vi "Main Test App.vi"() -> ()   [LabVIEW 2010]
panel:
  out "Limit Test Passed?":bool
  in  "Lower LED Limit (V)":dbl=1.63
  in  "Upper LED Limit (V)":dbl=1.635
  out "LED Test Passed?":bool
  in  "Filter Error Limits (+/- V)":dbl=0.06
  out "Limit Test Results":cluster{dbl[], dbl[]}[](graph)=[{[1000.0, 9166.666666666668, 17333.333333333336, 25500.0, 33666.66666666667, 41833.333333333336, 50000.0], [0.8109999999999999, 0.7375, 0.6639999999999999, 0.5905, 0.5169999999999999, 0.44349999999999995, 0.37]}, {[1000.0, 9166.666666666668, 17333.333333333336, 25500.0, 33666.66666666667, 41833.333333333336, 50000.0], [0.7794851199823166, 0.7105386097097423, 0.600359382509452, 0.5104585406834482, 0.4415120304108739, 0.3921679593334433, 0.3549909194805846]}, {[1000.0, 9166.666666666668, 17333.333333333336, 25500.0, 33666.66666666667, 41833.333333333336, 50000.0], [0.6910000000000001, 0.6174999999999999, 0.544, 0.4705, 0.39699999999999996, 0.32349999999999995, 0.25]}]
  in  "Select XML Config File":u16(ring)=2 items=["PXI Mod Instr Config 081226.xml", "Legacy Instr Config 081226.xml", "Simulated Instruments.xml"]
  out "Actual LED Voltage (V)":dbl
  in  "error in (no error)":errorcluster
  out "error out":errorcluster
  in  "Number of Steps":i32=7
  in  "Start Frequency (>1K Hz)":dbl=1000.0
  in  "Stop Frquency (<50k Hz)":dbl=50000.0
  # "Filter Limit Test Results"
  # "Filter Limit Test Parameters"
  # "LED Test Parameters"
  # "LED Test Results"
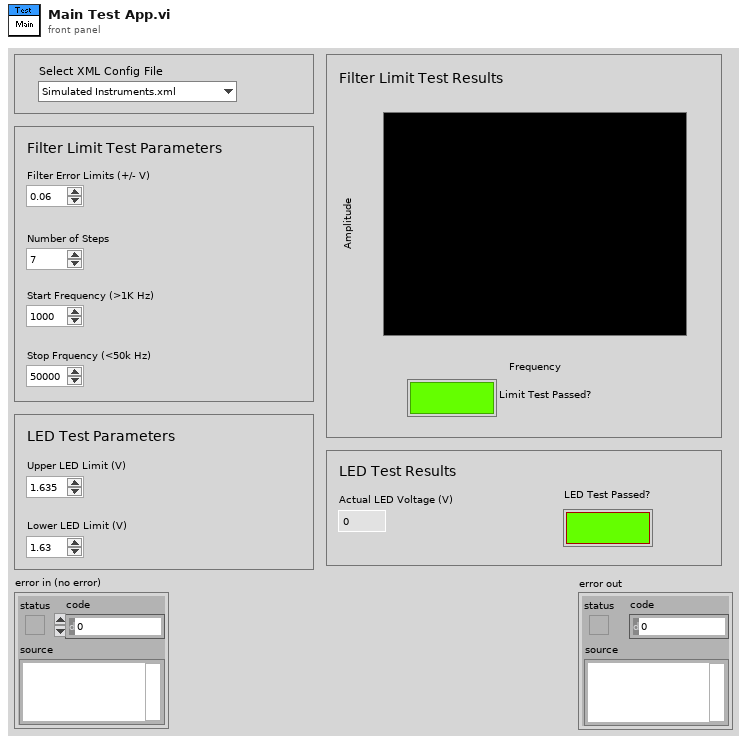
[diagram p1: front panel]
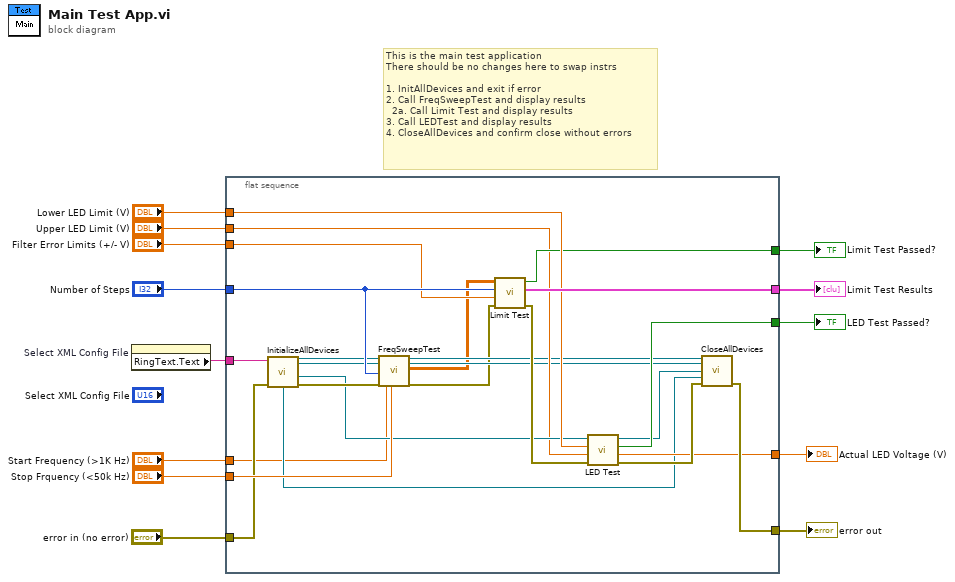
[diagram p0: block diagram]
diagram:
  # "This is the main test application\nThere should be no changes here to swap instrs\n\n1. InitAllDevices and exit if error\n2. Call FreqSweepTest and display results\n  2a. Call Limit Test and display results\n3. Call LEDTest and display results\n4. CloseAllDevices and confirm close without errors"
  n1 = property on="Select XML Config File" class="Ring (strict)"() -> ("RingText.Text"=w2:string)  [unwired: 2 in, 2 out]
  n2 = flat-sequence {
    tunnel: [w38] -> w13
    tunnel: "Stop Frquency (<50k Hz)" -> [w36]
    tunnel: "Number of Steps" -> [w35]
    tunnel: "Filter Error Limits (+/- V)" -> [w34]
    tunnel: [w33] -> w9
    tunnel: "Lower LED Limit (V)" -> [w31]
    tunnel: [w30] -> w7
    tunnel: [w26] -> w6
    tunnel: [w25] -> w5
    tunnel: "Upper LED Limit (V)" -> [w23]
    tunnel: "error in (no error)" -> [w18]
    tunnel: w2 -> [w17]
    tunnel: "Start Frequency (>1K Hz)" -> [w15]
    frame #0 {
      n3 = call "InitializeAllDevices.vi"("error in (no error)"=w18, "XML File Name"=w17) -> ("error out"=w27:errorcluster, "Meter"=w24:refnum<class "Meter.lvclass">, "Scope"=w28:refnum<class "Scope.lvclass">, "Signal Generator"=w29:refnum<class "Signal Generation.lvclass">, "Switch"=w16:refnum<class "Switch.lvclass">)  [unwired: 5 in]
      n4 = call "FreqSweepTest.vi"("Signal Generator"=w29, "Scope"=w28, "Number of Steps (25)"=w35, "error in (no error)"=w27, "Start Frequency (1000)"=w15, "Stop Frequency (50000)"=w36) -> ("Signal Generator Out"=w21:refnum<class "Signal Generation.lvclass">, "Scope Out"=w20:refnum<class "Scope.lvclass">, "Freq Amp Array"=w19:dbl[][], "error out"=w14:errorcluster)  [unwired: 10 in]
      n5 = call "Limit Test.vi"("error in (no error)"=w14, "Filter Error Limits"=w34, "Number of Steps"=w35, "Freq Amp Array"=w19) -> ("error out"=w32:errorcluster, "Limit Test Results"=w33:cluster{dbl[], dbl[]}[], "Test Passed?"=w30:bool)  [unwired: 1 in, 4 out]
      n6 = call "LED Test.vi"("error in (no error)"=w32, "Lower LED Limit (V)"=w23, "Upper LED Limit (V)"=w31, "Meter"=w24) -> ("error out"=w37:errorcluster, "Diode Voltage"=w25:dbl, "LED Test Passed?"=w26:bool, "Meter Out"=w22:refnum<class "Meter.lvclass">)  [unwired: 4 out]
      n7 = call "CloseAllDevices.vi"("Signal Generator"=w21, "Scope"=w20, "Meter"=w22, "Switch"=w16, "error in (no error)"=w37) -> ("error out"=w38:errorcluster)  [unwired: 10 in]
    }
  }
  "error out" <- w13
  "Actual LED Voltage (V)" <- w5
  "Limit Test Results" <- w9
  "LED Test Passed?" <- w6
  "Limit Test Passed?" <- w7
